vi "getKeyOrIndex2(30-03-2017).vi"(8 "error in (no error)":errorcluster, 9 "before match":string, 10 "previous level cluster":variant, 11 "input string":string) -> (0 "error out":errorcluster, 1 "value":string, 2 "key":string, 3 "index out":i32, 4 "error?":bool, 5 "Array Element":variant)   [LabVIEW 2015]
uses:
  <vilib>/regexp/Match Regular Expression.xnode
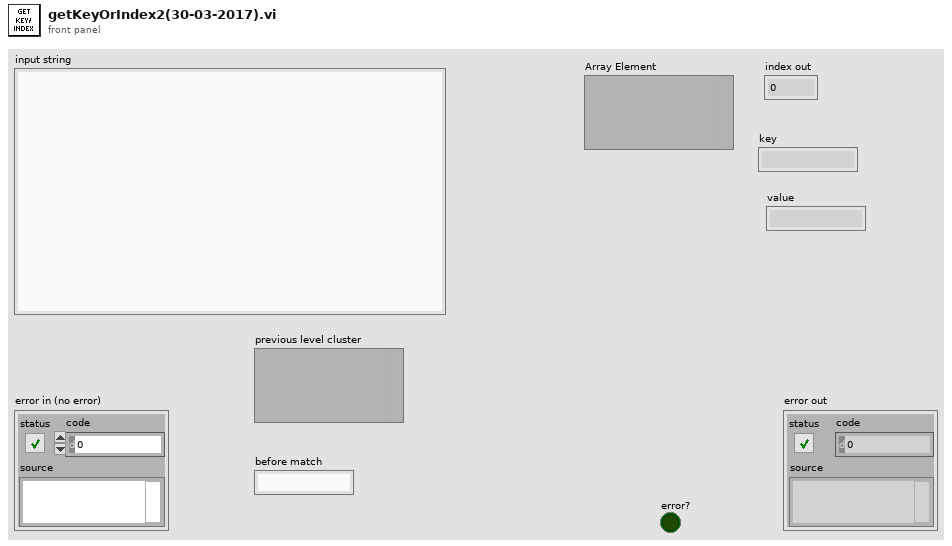
[diagram p1: front panel]
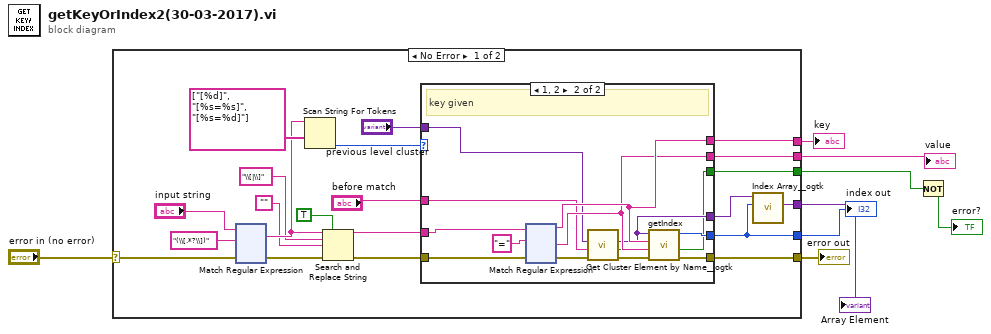
[diagram p0: block diagram]
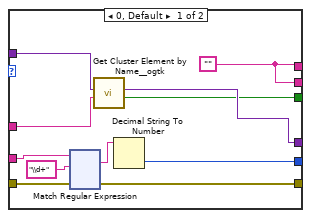
[diagram p2: hidden frame]
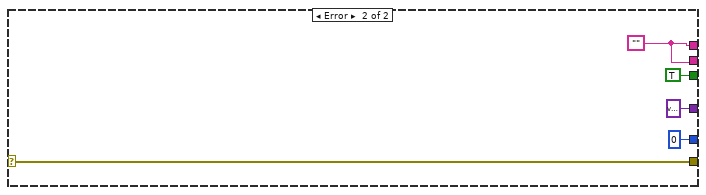
[diagram p3: hidden frame]
diagram:
  n1 = case shown="No Error" "error in (no error)" {
    selector: "error in (no error)" -> [w18 w400]
    tunnel: [w17 w400] -> w7
    tunnel: [w13 0 ("indexOut")] -> w6
    tunnel: [w16 w398] -> w5
    tunnel: [w15 w398] -> w4
    tunnel: [w12 variant ("Array Element")] -> w3
    tunnel: [w9 TRUE ("found?")] -> w2
    frame No Error {
      n2 = xnode "Match Regular Expression"("input string"="input string", "regular expression"="(\\[.*?\\])", "error in"=w18) -> ("whole match"=w26:string, "error out"=w19:errorcluster)  [unwired: 3 in, 3 out]
      n3 = Scan String For Tokens(7:string[] ["[%d]", "[%s=%s]", "[%s=%d]"] ("operators (none)"), 9:w26) -> (0:w21:i32)  [unwired: 4 in, 3 out]
      n4 = Search and Replace String(replace all?=TRUE ("replace all? (F)"), input string=w26, search string="\\[|\\]", replace string="", error in=w19) -> (result string=w23:string, error out=w20:errorcluster)  [unwired: 3 in, 2 out]
      n5 = case shown="1, 2" w21 {
        tunnel: w23 -> [w40 w167]
        tunnel: w20 -> [w37 w165]
        tunnel: [w36 w164] -> w13
        tunnel: [w35 w161] -> w17
        tunnel: [w34 w160] -> w16
        tunnel: [w34 w159] -> w15
        tunnel: [w31 w158] -> w14
        tunnel: "before match" -> [w32 w157]
        tunnel: "previous level cluster" -> [w33 w156]
        tunnel: [w30 w155] -> w9
        frame 0, Default {
          w34 = ""
          n6 = xnode "Match Regular Expression"("input string"=w40, "regular expression"="\\d+", "error in"=w37) -> ("whole match"=w38:string, "error out"=w35:errorcluster)  [unwired: 3 in, 3 out]
          n7 = call <userlib>:"Get Cluster Element by Name__ogtk.vi"("Element Name"=w32, "Cluster"=w33) -> ("found?"=w30:bool, "VElement"=w31:variant)  [unwired: 7 in, 1 out]
          n8 = Decimal String To Number(string=w38) -> (number=w36:i32)  [unwired: 2 in, 1 out]
        }
        frame 1, 2 {
          # "key given"
          n9 = xnode "Match Regular Expression"("input string"=w167, "regular expression"="=", "error in"=w165) -> ("before match"=w160:string, "after match"=w159:string, "error out"=w163:errorcluster)  [unwired: 3 in, 2 out]
          n10 = call <userlib>:"Get Cluster Element by Name__ogtk.vi"("error in (no error)"=w163, "Element Name"=w157, "Cluster"=w156) -> ("error out"=w162:errorcluster, "found?"=w155:bool, "VElement"=w158:variant)  [unwired: 6 in]
          n11 = call "getIndex.vi"("error in (no error)"=w162, "value"=w159, "key"=w160, "VElement"=w158) -> ("error out"=w161:errorcluster, "indexOut"=w164:i32)  [unwired: 6 in]
        }
      }
      n12 = call <userlib>:"Index Array__ogtk.vi"("Index (1D)"=w13, "MultiD Array"=w14) -> ("Array Element"=w12:variant)  [unwired: 8 in, 1 out]
    }
    frame Error {
      w398 = ""
    }
  }
  "error out" <- w7
  "index out" <- w6
  "key" <- w5
  "value" <- w4
  "Array Element" <- w3
  n13 = Not(x=w2) -> (.not. x?=→"error?":bool)
